vi "FGV Referenzen.vi"(5 "Aktikon":enum16{"lesen", "schreiben"}(ring), 7 "error in (no error)":errorcluster caption="Fehler (Eingang, kein Fehler)", 10 "Referenzen Cluster in":T1) -> (0 "error out":errorcluster caption="Fehler (Ausgang)", 3 "Referenzen Cluster out":T1)   [LabVIEW 2020, in "Linearisierung v2.lvlib" / "Protokoll.lvlib"]
uses:
  Protokoll.lvlib
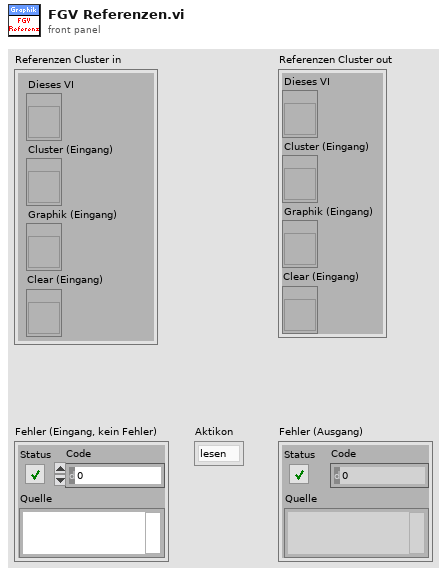
[diagram p1: front panel]
types:
  T1 = cluster{"Dieses VI":refnum<vi>, "Cluster (Eingang)":refnum<vi>, "Graphik (Eingang)":refnum<vi>, "Clear (Eingang)":refnum<vi>}
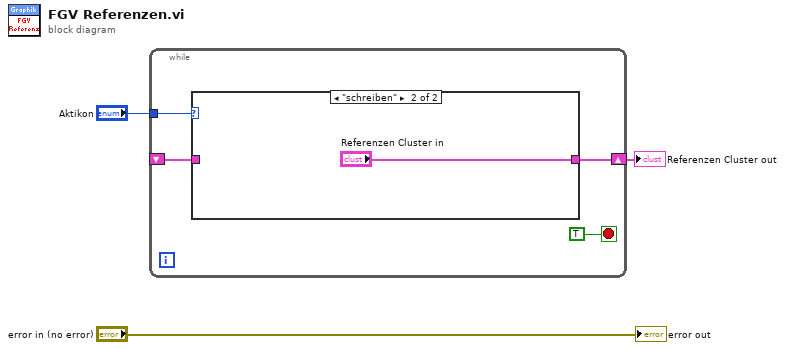
[diagram p0: block diagram]
diagram:
  n1 = while {
    tunnel: "Aktikon" -> [w7]
    shift-right: [w5] -> w2
    shift-left: _ -> [w4]
    stop <- TRUE stop-if-true
    n2 = case shown="\"schreiben\"" w7 {
      tunnel: [w8 "Referenzen Cluster in"] -> w5
      tunnel: w4 -> [w8 _]
      frame "lesen", Default {
      }
      frame "schreiben" {
      }
    }
  }
  "Referenzen Cluster out" <- w2
  "error out" <- "error in (no error)"
